vi "军蚁-启用菜单功能.vi"(8 "error in":errorcluster caption="error out", 10 "数组":bool[](array[boolean])=[TRUE, TRUE, TRUE, TRUE, TRUE, TRUE, TRUE, TRUE], 11 "菜单引用":refnum<k9>) -> (0 "error out":errorcluster)   [LabVIEW 2017]
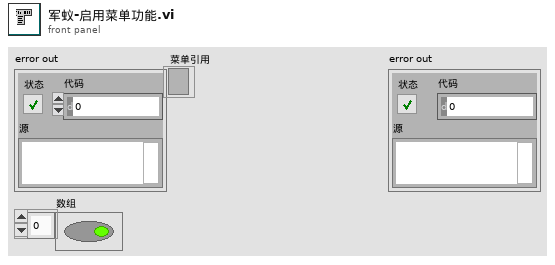
[diagram p1: front panel]
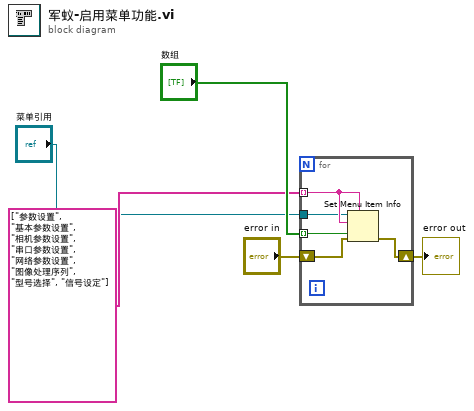
[diagram p0: block diagram]
diagram:
  n1 = for {
    tunnel: string[] ["参数设置", "基本参数设置", "相机参数设置", "串口参数设置", "网络参数设置", "图像处理序列", "型号选择", "信号设定"] -> [w10] mode=indexing
    tunnel: "数组" -> [w9] mode=indexing
    shift-right: [w8] -> w2
    shift-left: "error in" -> [w7]
    tunnel: "菜单引用" -> [w6]
    n2 = Set Menu Item Info(7:w10, 8:w7, 9:w9, 10:w10, 11:w6) -> (0:w8:errorcluster)  [unwired: 2 in, 1 out]
  }
  "error out" <- w2
